vi "updateStadisticDataInStadisticTable.vi"(8 "error in":errorcluster, 11 "dataReadingToUpdate":T2) -> (0 "error out":errorcluster, 3 "dataUpdate":T1)   [LabVIEW 2014]
uses:
  <vilib>/addons/database/NI_Database_API.lvlib
  <vilib>/addons/database/Connection.llb/DB Tools Open Connec (String).vi
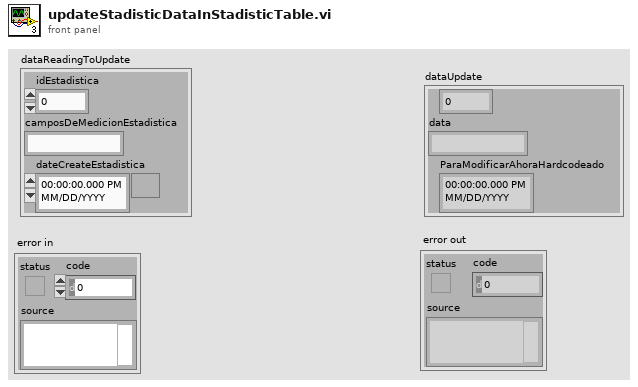
[diagram p1: front panel]
types:
  T1 = cluster{dbl, "data":string, "ParaModificarAhoraHardcodeado":timestamp}
  T2 = cluster{"idEstadistica":dbl, "camposDeMedicionEstadistica":string, "dateCreateEstadistica":timestamp}
  T3 = typedef "NI_Database_API.lvlib/Conn ObjectReference.ctl" = refnum<k1>
  T4 = typedef "NI_Database_API.lvlib/DB Tools DataTypes.ctl" = enum16{"String", "Long (I32)", "Single (SGL)", "Double (DBL)", "Date/Time", "Binary"}
  T5 = cluster{"name":string, "database data type":T4, "defined size":i32}[]
  T6 = cluster{cluster{string, string, string, string, string}, string[]}
  T7 = cluster{cluster{string, string, string}, string[]}
  T8 = cluster{"idProducto":dbl, "outDiameterProducto":string, "steelGradeProducto":string, "loteProducto":string, "dateCreateProducto":timestamp, "idRecipe":dbl}
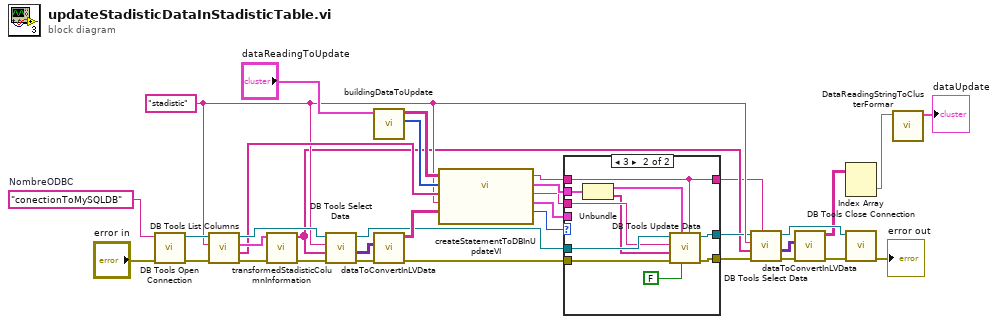
[diagram p0: block diagram]
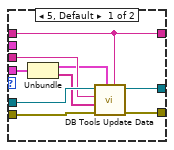
[diagram p2: hidden frame]
diagram:
  w11 = "stadistic" ("tableName")
  w35 = "conectionToMySQLDB"  # NombreODBC
  n1 = call-poly <vilib>:"DB Tools Open Connection.vi"("error in (no error)"="error in", "connection information"=w35) -> ("error out"=w32:errorcluster, "connection reference"=w33:T3)  [unwired: 6 in]
  n2 = call <vilib>:"DB Tools List Columns.vi"("error in (no error)"=w32, "table"=w11, "connection reference"=w33) -> ("error out"=w30:errorcluster, "columns"=w18:string[], "column information"=w31:T5, "connection reference out"=w29:T3)  [unwired: 1 in]
  n3 = call "transformedStadisticColumnInformation.vi"("error in"=w30, "columnInformationReading"=w31) -> ("error out"=w28:errorcluster, "columnInformationReadingTransformed"=w9:string[])  [unwired: 8 in]
  n4 = call <vilib>:"DB Tools Select Data.vi"("error in (no error)"=w28, "columns"=w9, "table"=w11, "connection reference"=w29) -> ("error out"=w27:errorcluster, "data"=w26:variant[][], "connection reference out"=w16:T3)  [unwired: 2 in]
  n5 = call "buildingDataToUpdate.vi"("dataReadingToUpdate"="dataReadingToUpdate") -> ("RawIndexToModifyOut"=w13:i32[], "ItemNamesOut"=w14:string[][])  [unwired: 9 in]
  n6 = call "dataToConvertInLVData.vi"("error in"=w27, "dataReadingIn"=w26) -> ("error out"=w17:errorcluster, "dataReadingOut"=w19:string[][])  [unwired: 8 in]
  n7 = call "createStatementToDBInUpdateVI.vi"("DataReadingInTableBeforeToUpdate"=w19, "Nombre Tabla"=w11, "ColumnName"=w18, "RawIndexToModify"=w13, "ItemNames"=w14) -> ("DataToModify5"=w23:T6, "TableNameToModify"=w22:string, "DataToModify3"=w24:T7, "statementSQL"=w25:string, "NumberOfFields"=w21:i32)  [unwired: 2 in]
  n8 = case shown="3" w21 {
    tunnel: w16 -> [w41 w54]
    tunnel: w17 -> [w42 w53]
    tunnel: [w43 w52] -> w10
    tunnel: [w44 w51] -> w12
    tunnel: w22 -> [w40 w50]
    tunnel: w25 -> [w36 w45]
    tunnel: w24 -> [_ w48]
    tunnel: w23 -> [w39 _]
    tunnel: [w36 w45] -> w8
    frame 5, Default {
      n9 = Unbundle(w39) -> (w38:cluster{string, string, string, string, string}, w37:string[])
      n10 = call <vilib>:"DB Tools Update Data.vi"("condition"=w36, "data"=w38, "error in (no error)"=w42, "columns"=w37, "table"=w40, "connection reference"=w41) -> ("error out"=w44:errorcluster, "connection reference out"=w43:T3)  [unwired: 4 in]
    }
    frame 3 {
      n11 = Unbundle(w48) -> (w47:cluster{string, string, string}, w46:string[])
      n12 = call <vilib>:"DB Tools Update Data.vi"("condition"=w45, "flatten cluster? (F)"=FALSE, "data"=w47, "error in (no error)"=w53, "columns"=w46, "table"=w50, "connection reference"=w54) -> ("error out"=w51:errorcluster, "connection reference out"=w52:T3)  [unwired: 3 in]
    }
  }
  n13 = call <vilib>:"DB Tools Select Data.vi"("condition"=w8, "error in (no error)"=w12, "columns"=w9, "table"=w11, "connection reference"=w10) -> ("error out"=w4:errorcluster, "data"=w5:variant[][], "connection reference out"=w7:T3)  [unwired: 1 in]
  n14 = call "dataToConvertInLVData.vi"("error in"=w4, "dataReadingIn"=w5) -> ("error out"=w3:errorcluster, "dataReadingOut"=w6:string[][])  [unwired: 8 in]
  n15 = Index Array(array=w6) -> (element=w2:string[])  [unwired: 2 in]
  n16 = call <vilib>:"DB Tools Close Connection.vi"("error in (no error)"=w3, "connection reference"=w7) -> ("error out"=→"error out":errorcluster)  [unwired: 5 in]
  n17 = call "DataReadingStringToClusterFormar.vi"("StringFormat"=w2) -> ("ClusterFormat"=→"dataUpdate":T8)  [unwired: 10 in]
